vi "Snapshot_noCall.vi"(6 "Dest Format":string(combo)="{6fddc324-4e03-4bfe-b185-3d77768dc90e}", 11 "WebBrowser":refnum<k24>) -> ()   [LabVIEW 2016]
uses:
  System.Windows.Forms
  <vilib>/vision/Image Controls.llb/IMAQ Image.ctl
panel:
  out "string 2":string
  out "Dest Format":string(combo)="{6fddc324-4e03-4bfe-b185-3d77768dc90e}"
  out "Image":T1(plugin-control)
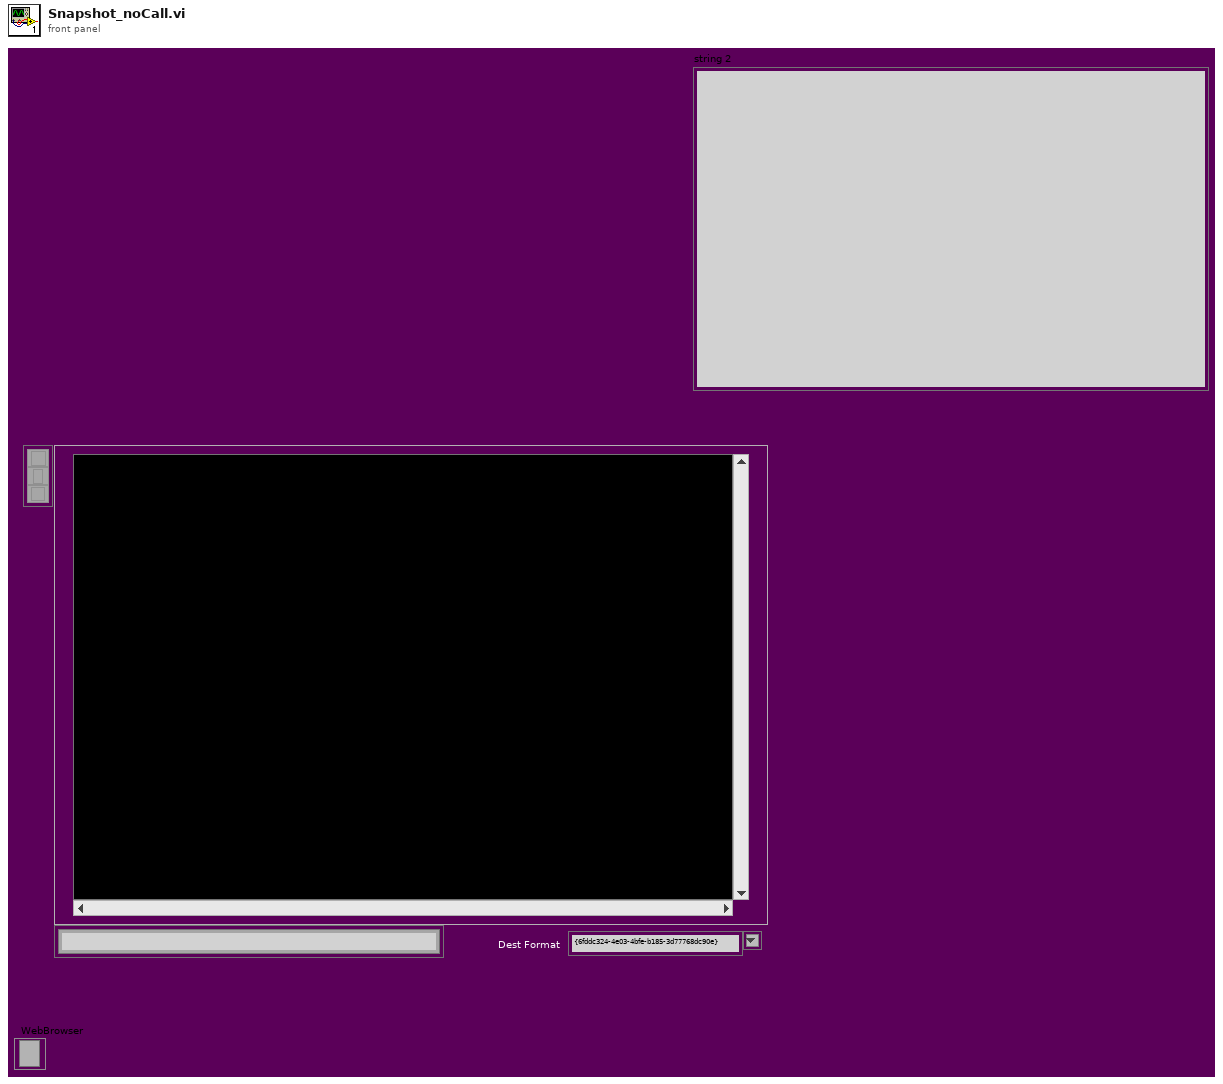
[diagram p1: front panel]
types:
  T1 = typedef "IMAQ Image.ctl" = refnum<image>
  T2 = typedef "Image Type" = u32
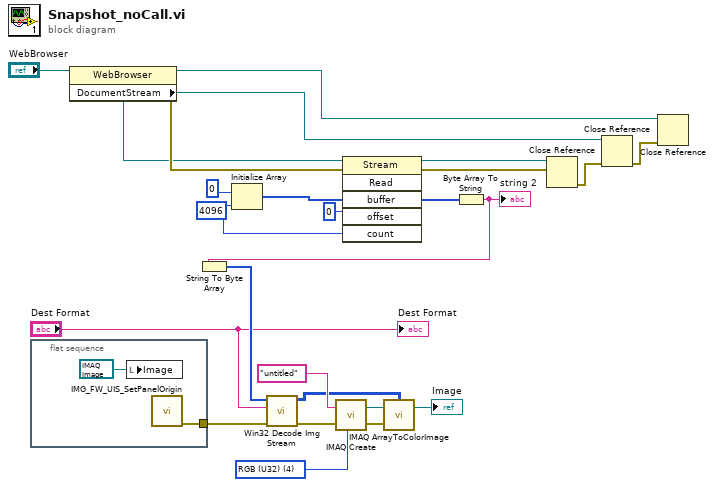
[diagram p0: block diagram]
diagram:
  w11 = 4096 ("dimension size")
  w23 = T2 4 items=["Grayscale (U8)", "Grayscale (I16)", "Grayscale (SGL)", "Complex (CSG)", "RGB (U32)", "HSL (U32)", "RGB (U64)", "Grayscale (U16)"] ("Image Type")
  n1 = flat-sequence {
    tunnel: [w25] -> w15
    frame #0 {
      n2 = local write "Image"(T1 refnum ("New Image")) -> ()
      n3 = call "IMG_FW_UIS_SetPanelOrigin.vi"() -> ("error out"=w25:errorcluster)  [unwired: 11 in]
    }
  }
  n4 = property class="WebBrowser"(reference="WebBrowser") -> (reference out=w1:refnum<k24>, error out=w3:errorcluster, "DocumentStream"=w2:refnum<k24>)  [unwired: 1 in]
  n5 = Initialize Array(u8 0, w11) -> (w13:u8[])
  n6 = invoke class="Stream" method="Read"(reference=w2, error in=w3, "buffer"=w13, "offset"=0, "count"=w11) -> (reference out=w9:refnum<k24>, error out=w6:errorcluster, "buffer"=w10:u8[])  [unwired: 1 in, 3 out]
  n7 = Byte Array To String(unsigned byte array=w10) -> (string=w5:string)
  "string 2" <- w5
  n8 = String To Byte Array(string=w5) -> (unsigned byte array=w21:u8[])
  n9 = call "Win32 Decode Img Stream.vi"("error in (no error)"=w15, "Dest Format"="Dest Format", "Image Data"=w21) -> ("error out"=w18:errorcluster, "Dest"=w20:u32[][])  [unwired: 4 in, 3 out]
  n10 = call "IMAQ Create"("Image Name"="untitled", "Image Type"=w23, "error in (no error)"=w18) -> ("New Image"=w24:T1, "error out"=w19:errorcluster)  [unwired: 2 in]
  n11 = call "IMAQ ArrayToColorImage"("Image Pixels (U32)"=w20, "Image"=w24, "error in (no error)"=w19) -> ("Image Out"=→"Image":T1)  [unwired: 2 in, 1 out]
  n12 = Close Reference(reference=w9, error in (no error)=w6) -> (error out=w8:errorcluster)
  n13 = Close Reference(reference=w2, error in (no error)=w8) -> (error out=w7:errorcluster)
  n14 = Close Reference(reference=w1, error in (no error)=w7) -> ()  [unwired: 1 out]
  "Dest Format" <- "Dest Format"
